vi "53230A_Freq_Counter_Measure_Configure(Freq & Duty Cycle).vi"(0 "VISA resource name":refnum<visa-resource-name>, 1 "Measure":enum16{"Frequency", "Duty Cycle"}(ring), 2 "Channel (1:Channel 1)":i32(ring)=1 items=["Channel 1"=1, "Channel 2"=2, "Channel 3"=3], 3 "Sample Count (1)":i32=5, 4 "Gate Source (0: Time)":i32(ring) items=["Time", "External", "Input1", "Input2", "Advanced"], 5 "error in (no error)":errorcluster, 6 "Operation":enum16{"Configure", "Measure"}(ring)=enum."Measure", 7 "Timeout (10000 ms)":u32=10000, 8 "Reset (True)":bool, 9 "Statistics (ON/OFF)":bool=TRUE, 10 "ID Query (True)":bool, 11 "Enable Filter (F: Disable)":bool=TRUE, 13 "Time Resolution (0.1 s)":dbl=0.1 format="%#_6p") -> (14 "VISA resource name out":refnum<visa-resource-name>, 16 "Measurement":T1 {"Allan_Dev" format="%#_12g"; "Maximum" format="%#_12g"; "Minimum" format="%#_12g"; "Mean" format="%#_12g"}, 18 "status":bool, 19 "error out":errorcluster)   [LabVIEW 2016]
uses:
  <userlib>/_TI-LA/Instr Drivers/Counter/E532XX/Driver/Base/Public/Configure/Configure Channel (Basic).vi
  <userlib>/_TI-LA/Instr Drivers/Counter/E532XX/Driver/Base/Public/Configure/Measurement/Configure Measurement (Frequency).vi
  <userlib>/_TI-LA/Instr Drivers/Counter/E532XX/Driver/Base/Public/Configure/Measurement/Configure Measurement (Duty Cycle).vi
  <userlib>/_TI-LA/Instr Drivers/Counter/E532XX/Driver/Base/Public/Data/Low Level/Fetch Measurement (Statistics).vi
  <userlib>/_TI-LA/Instr Drivers/Counter/E532XX/Driver/Base/Agilent 532XX Series.lvlib
panel:
  in  "Tab Control":enum32{"Config", "Measure"}(tab)
  out "Execution Time":u32
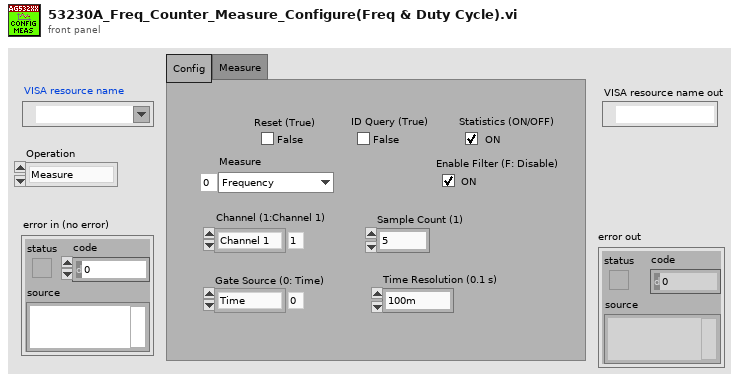
[diagram p1: front panel]
types:
  T1 = cluster{"Mean":dbl, "SDEV":dbl, "Minimum":dbl, "Maximum":dbl, "Allan_Dev":dbl}
  T2 = cluster{"Mean":dbl, "Standard Deviation":dbl, "Minimum":dbl, "Maximum":dbl, "Allan_Dev":dbl}
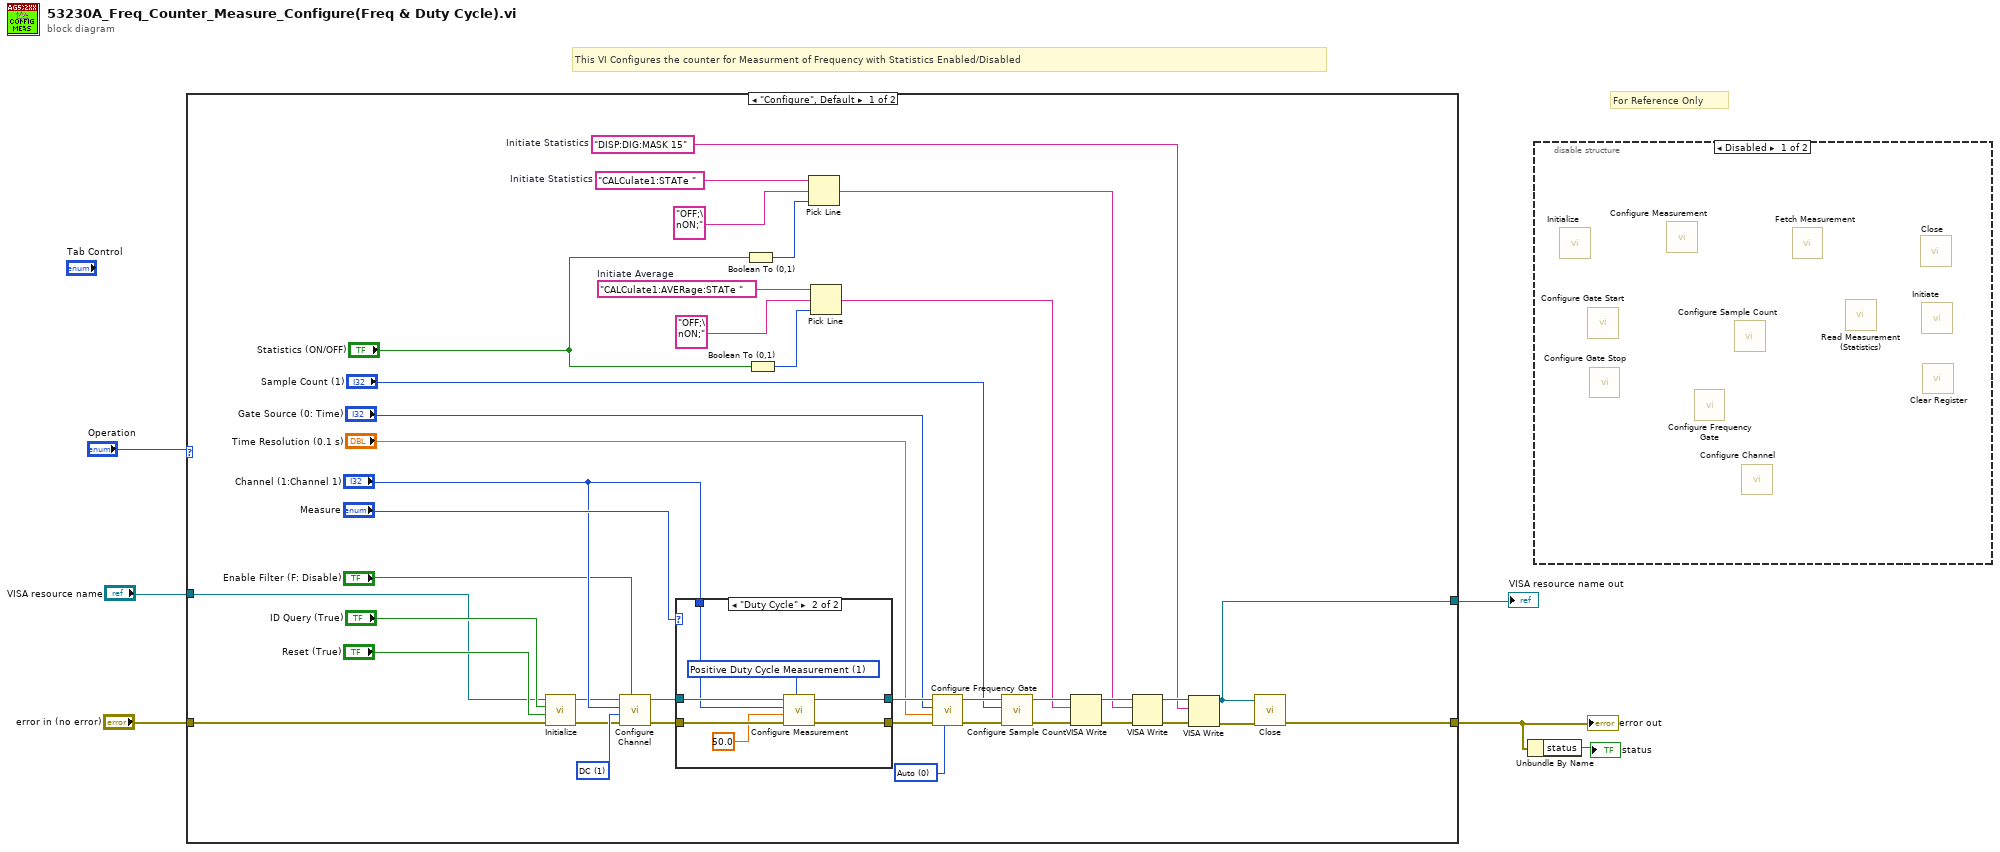
[diagram p0: block diagram]
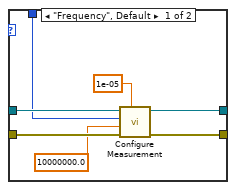
[diagram p2: hidden frame]
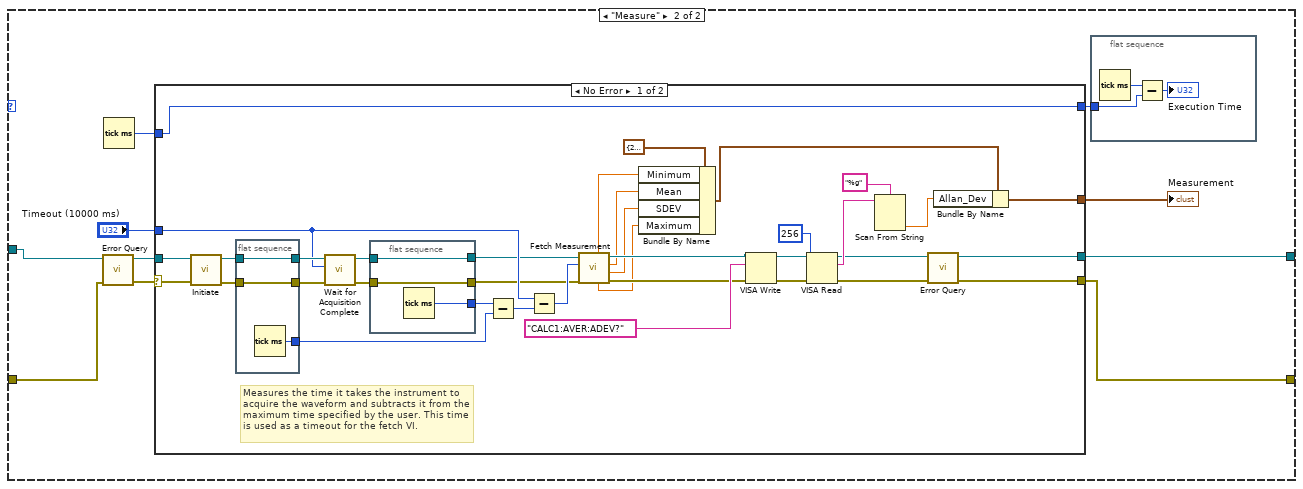
[diagram p3: hidden frame]
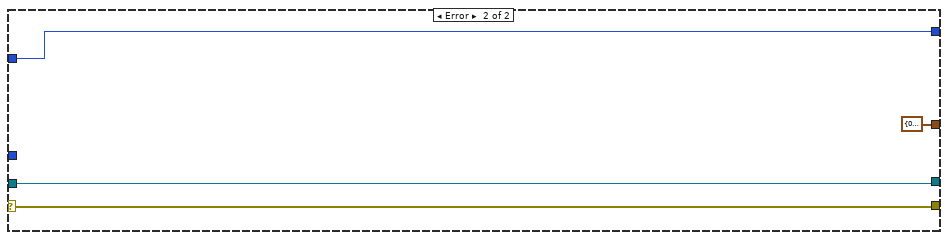
[diagram p4: hidden frame]
diagram:
  # "For Reference Only"
  # "This VI Configures the counter for Measurment of Frequency with Statistics Enabled/Disabled"
  n1 = case shown="\"Configure\", Default" "Operation" {
    tunnel: [w33 w63] -> w3
    tunnel: "VISA resource name" -> [w10 w62]
    tunnel: "error in (no error)" -> [w9 w61]
    tunnel: [w8 w64] -> w2
    frame "Configure", Default {
      w13 = 1 items=["AC", "DC"] ("Coupling (0: AC)")
      w18 = "DISP:DIG:MASK 15"  # Initiate Statistics
      w26 = "CALCulate1:STATe "  # Initiate Statistics
      w32 = "CALCulate1:AVERage:STATe "  # Initiate Average
      w39 = 0 items=["Auto", "Reciprocal", "Continuous"] ("Measurement Mode (0: Auto)")
      n2 = call <userlib>:"Initialize.vi"("error in (no error)"=w9, "Reset (True)"="Reset (True)", "ID Query (True)"="ID Query (True)", "VISA resource name"=w10) -> ("error out"=w11:errorcluster, "VISA resource name out"=w12:refnum<visa-resource-name>)  [unwired: 6 in]
      n3 = call-poly <userlib>:"Configure Channel.vi"("Enable Filter (F: Disable)"="Enable Filter (F: Disable)", "error in (no error)"=w11, "Coupling (0: AC)"=w13, "Channel (1: Channel 1)"="Channel (1:Channel 1)", "VISA resource name"=w12) -> ("error out"=w15:errorcluster, "VISA resource name out"=w16:refnum<visa-resource-name>)  [unwired: 5 in]
      n4 = case shown="\"Duty Cycle\"" "Measure" {
        tunnel: w16 -> [w52 w59]
        tunnel: w15 -> [w51 w58]
        tunnel: "Channel (1:Channel 1)" -> [w50 w55]
        tunnel: [w47 w56] -> w43
        tunnel: [w46 w57] -> w42
        frame "Frequency", Default {
          n5 = call-poly <userlib>:"Configure Measurement.vi"("Frequency Resolution (1 Hz)"=1e-05, "error in (no error)"=w51, "Frequency Estimate (10E+6 Hz)"=10000000.0, "Channel (1:Channel 1)"=w50, "VISA resource name"=w52) -> ("error out"=w46:errorcluster, "VISA resource name out"=w47:refnum<visa-resource-name>)  [unwired: 5 in]
        }
        frame "Duty Cycle" {
          w53 = 1 items=["Negative Duty Cycle Measurement", "Positive Duty Cycle Measurement"] ("Duty Cycle Type (0: Negative Duty Cycle Measurement)")
          n6 = call-poly <userlib>:"Configure Measurement.vi"("Duty Cycle Type (0: Negative Duty Cycle Measurement)"=w53, "error in (no error)"=w58, "Signal Reference Level (50 Percent)"=50.0, "Channel (1: Channel 1)"=w55, "VISA resource name"=w59) -> ("error out"=w57:errorcluster, "VISA resource name out"=w56:refnum<visa-resource-name>)  [unwired: 5 in]
        }
      }
      n7 = Boolean To (0,1)(Boolean="Statistics (ON/OFF)") -> (0, 1=w28:i16)
      n8 = Boolean To (0,1)(Boolean="Statistics (ON/OFF)") -> (0, 1=w30:i16)
      n9 = Pick Line(string ("")=w26, multi-line string="OFF;\nON;", line index=w28) -> (output string=w22:string)
      n10 = Pick Line(string ("")=w32, multi-line string="OFF;\nON;", line index=w30) -> (output string=w29:string)
      n11 = call <userlib>:"Configure Frequency Gate.vi"("Measurement Mode (0: Auto)"=w39, "error in (no error)"=w42, "Time Resolution (0.1 s)"="Time Resolution (0.1 s)", "Gate Source (0: Time)"="Gate Source (0: Time)", "VISA resource name"=w43) -> ("error out"=w36:errorcluster, "VISA resource name out"=w37:refnum<visa-resource-name>)  [unwired: 5 in]
      n12 = call <userlib>:"Configure Sample Count.vi"("error in (no error)"=w36, "Sample Count (1)"="Sample Count (1)", "VISA resource name"=w37) -> ("error out"=w35:errorcluster, "VISA resource name out"=w38:refnum<visa-resource-name>)  [unwired: 7 in]
      n13 = VISA Write(VISA resource name=w38, write buffer=w29, error in (no error)=w35) -> (VISA resource name out=w23:refnum<visa-resource-name>, error out=w24:errorcluster)  [unwired: 1 out]
      n14 = VISA Write(VISA resource name=w23, write buffer=w22, error in (no error)=w24) -> (VISA resource name out=w20:refnum<visa-resource-name>, error out=w21:errorcluster)  [unwired: 1 out]
      n15 = VISA Write(VISA resource name=w20, write buffer=w18, error in (no error)=w21) -> (VISA resource name out=w8:refnum<visa-resource-name>, error out=w19:errorcluster)  [unwired: 1 out]
      n16 = call <userlib>:"Close.vi"("error in (no error)"=w19, "VISA resource name"=w8) -> ("error out"=w33:errorcluster)  [unwired: 9 in]
    }
    frame "Measure" {
      n17 = call <userlib>:"Error Query.vi"("error in (no error)"=w61, "VISA resource name"=w62) -> ("error out"=w67:errorcluster, "VISA resource name out"=w66:refnum<visa-resource-name>)  [unwired: 8 out]
      n18 = Tick Count (ms)() -> (millisecond timer value=w68:u32)
      n19 = case shown="No Error" w67 {
        selector: w67 -> [w82 w118]
        tunnel: [w108 w117] -> w64
        tunnel: "Timeout (10000 ms)" -> [w101 _]
        tunnel: [w94 w118] -> w63
        tunnel: w66 -> [w83 w117]
        tunnel: w68 -> [w81 w116]
        tunnel: [w81 w116] -> w69
        tunnel: [w80 T2 {"Mean"=0.0, "Standard Deviation"=0.0, "Minimum"=0.0, "Maximum"=0.0, "Allan_Dev"=0.0} ("Measure")] -> w60
        frame No Error {
          # "Measures the time it takes the instrument to acquire the waveform and subtracts it from the maximum time specified by the user. This time is used as a timeout for the fetch VI."
          n20 = call <userlib>:"Initiate.vi"("error in (no error)"=w82, "VISA resource name"=w83) -> ("error out"=w105:errorcluster, "VISA resource name out"=w106:refnum<visa-resource-name>)  [unwired: 8 out]
          n21 = flat-sequence {
            tunnel: [w114] -> w102
            tunnel: w106 -> [w114]
            tunnel: [w113] -> w103
            tunnel: w105 -> [w113]
            tunnel: [w112] -> w104
            frame #0 {
              n22 = Tick Count (ms)() -> (millisecond timer value=w112:u32)
            }
          }
          n23 = call <userlib>:"Wait for Acquisition Complete.vi"("error in (no error)"=w103, "Maximum Time (10000 ms)"=w101, "VISA resource name"=w102) -> ("error out"=w99:errorcluster, "VISA resource name out"=w100:refnum<visa-resource-name>)  [unwired: 1 in, 6 out]
          n24 = flat-sequence {
            tunnel: [w111] -> w95
            tunnel: w100 -> [w111]
            tunnel: [w110] -> w96
            tunnel: w99 -> [w110]
            tunnel: [w109] -> w98
            frame #0 {
              n25 = Tick Count (ms)() -> (millisecond timer value=w109:u32)
            }
          }
          n26 = Subtract(x=w98, y=w104) -> (x-y=w107:u32)
          n27 = Subtract(x=w101, y=w107) -> (x-y=w97:u32)
          n28 = call-poly <userlib>:"Fetch Measurement.vi"("error in (no error)"=w96, "Timeout (10000 ms)"=w97, "VISA resource name"=w95) -> ("error out"=w86:errorcluster, "Standard Deviation"=w74:dbl, "Mean"=w75:dbl, "VISA resource name out"=w87:refnum<visa-resource-name>, "Maximum"=w76:dbl, "Minimum"=w73:dbl)  [unwired: 3 out]
          n29 = Bundle By Name(cluster=T1 {"Mean"=29999993.2162221, "SDEV"=0.0613282167045458, "Minimum"=29999993.1086075, "Maximum"=29999993.2937739, "Allan_Dev"=0.0363360449059443} ("Measure"), "Minimum"=w73, "Mean"=w75, "SDEV"=w74, "Maximum"=w76) -> (w78:T1)
          n30 = VISA Write(VISA resource name=w87, write buffer="CALC1:AVER:ADEV?", error in (no error)=w86) -> (VISA resource name out=w92:refnum<visa-resource-name>, error out=w91:errorcluster)  [unwired: 1 out]
          n31 = VISA Read(VISA resource name=w92, byte count=u32 256, error in (no error)=w91) -> (VISA resource name out=w84:refnum<visa-resource-name>, read buffer=w89:string, error out=w85:errorcluster)  [unwired: 1 out]
          n32 = Scan From String(format string="%g", input string=w89) -> (output 1=w77:dbl)  [unwired: 3 in, 3 out]
          n33 = call <userlib>:"Error Query.vi"("error in (no error)"=w85, "VISA resource name"=w84) -> ("error out"=w94:errorcluster, "VISA resource name out"=w108:refnum<visa-resource-name>)  [unwired: 8 out]
          n34 = Bundle By Name(cluster=w78, "Allan_Dev"=w77) -> (w80:T1)
        }
        frame Error {
        }
      }
      "Measurement" <- w60
      n35 = flat-sequence {
        tunnel: w69 -> [w72]
        frame #0 {
          n36 = Tick Count (ms)() -> (millisecond timer value=w71:u32)
          n37 = Subtract(x=w71, y=w72) -> (x-y=→"Execution Time":u32)
        }
      }
    }
  }
  "error out" <- w3
  "VISA resource name out" <- w2
  n38 = Unbundle By Name(w3) -> ("status"=→"status":bool)
  n39 = disable-structure shown="Disabled" {
    frame Disabled {
      n40 = call <userlib>:"Initialize.vi"() -> ()  [unwired: 10 in, 2 out]
      n41 = call <userlib>:"Configure Gate Start.vi"() -> ()  [unwired: 10 in, 2 out]
      n42 = call <userlib>:"Configure Gate Stop.vi"() -> ()  [unwired: 10 in, 2 out]
      n43 = call-poly <userlib>:"Configure Measurement.vi"() -> ()  [unwired: 10 in, 2 out]
      n44 = call <userlib>:"Configure Frequency Gate.vi"() -> ()  [unwired: 10 in, 2 out]
      n45 = call <userlib>:"Configure Sample Count.vi"() -> ()  [unwired: 10 in, 2 out]
      n46 = call-poly <userlib>:"Configure Channel.vi"() -> ()  [unwired: 10 in, 2 out]
      n47 = call-poly <userlib>:"Fetch Measurement.vi"() -> ()  [unwired: 6 in, 6 out]
      n48 = call <userlib>:"Read Measurement (Statistics).vi"() -> ()  [unwired: 6 in, 6 out]
      n49 = call <userlib>:"Close.vi"() -> ()  [unwired: 11 in, 1 out]
      n50 = call <userlib>:"Initiate.vi"() -> ()  [unwired: 10 in, 2 out]
      n51 = call <userlib>:"Clear Register .vi"() -> ()  [unwired: 10 in, 2 out]
    }
    frame Enabled {
    }
  }
